vi "HTTPHeaderLine.vi"(8 "error in (no error)":errorcluster, 11 "HTTP Request Line":string) -> (0 "error out":errorcluster, 1 "Protocol":string, 2 "Request URI":string, 3 "Method":string)   [LabVIEW 2014, in "QwaveSys RPi Training Library.lvlib" / "WebSockets.lvlib"]
doc: "Parses the first line of the received HTTP headers (e.g. GET / HTTP/1.1)\nWebSockets API 1.3.0.13\nSam Sharp - Intelligent Energy\nCopyright (c) 2015, Intelligent Energy"
uses:
  <vilib>/Q-Wave Systems/QwaveSys RPi Training Package (Demo)/Addons/WebSockets API/WebSockets/WebSockets.lvlib
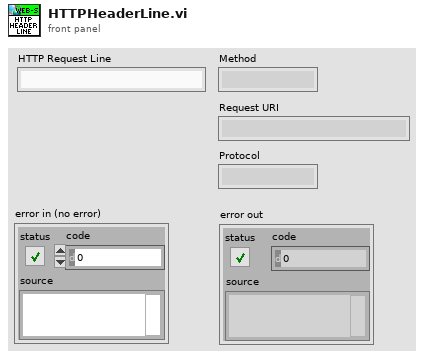
[diagram p1: front panel]
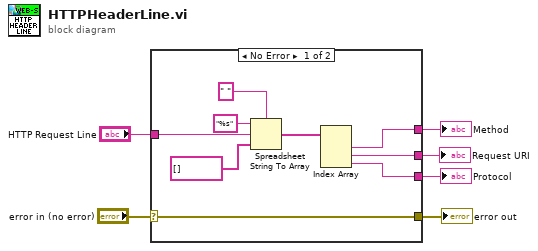
[diagram p0: block diagram]
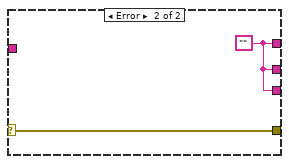
[diagram p2: hidden frame]
diagram:
  n1 = case shown="No Error" "error in (no error)" {
    selector: "error in (no error)" -> [w7 w17]
    tunnel: "HTTP Request Line" -> [w12 _]
    tunnel: [w10 w16] -> w5
    tunnel: [w9 w16] -> w4
    tunnel: [w8 w16] -> w3
    tunnel: [w7 w17] -> w1
    frame No Error {
      n2 = Spreadsheet String To Array(delimiter (Tab)=" ", format string="%s", spreadsheet string=w12, array type (2D Dbl)=string[] []) -> (array=w14:string[])
      n3 = Index Array(array=w14) -> (element #1=w9:string, element #2=w10:string, element #3=w8:string)  [unwired: 3 in]
    }
    frame Error {
      w16 = ""
    }
  }
  "Request URI" <- w5
  "Method" <- w4
  "Protocol" <- w3
  "error out" <- w1
